vi "State Description - HelperVI and Equivalent String.vi"() -> ()   [LabVIEW 2014]
uses:
  user.lib/_NEVSTOP/JKI State Machine ++/JKI-State-Machine-Plus.lvlib
panel:
  out "Equivalent String (Broadcast Message with Argument)":string="Status Changed >> Argument-> <all>"
  out "Equivalent String (Broadcast Message)":string="Status Changed-> <all>"
  out "Equivalent String (Async Message)":string="State >> Argument->DestModuleName"
  out "Equivalent String (Sync Message)":string="State >> Argument@DestModuleName"
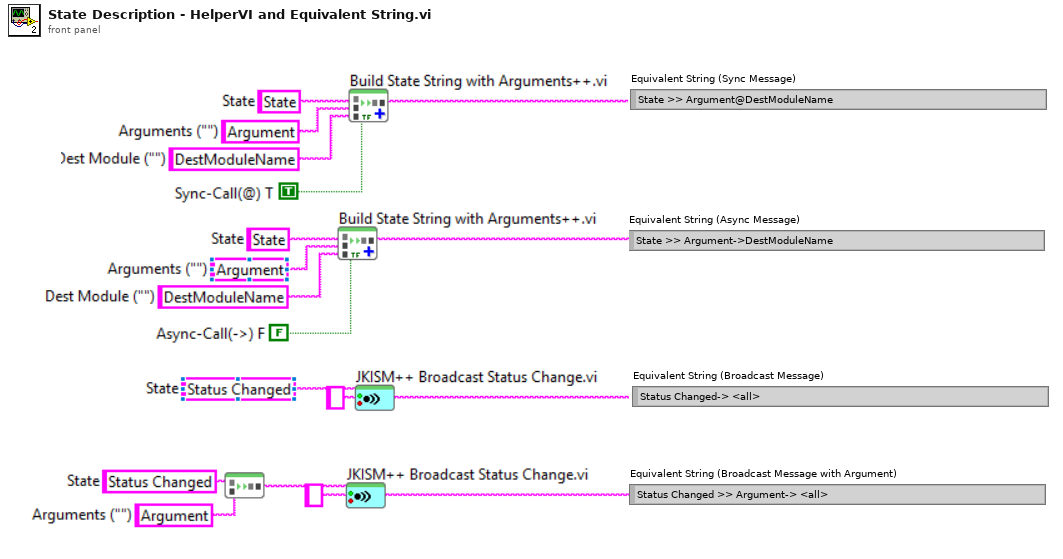
[diagram p1: front panel]
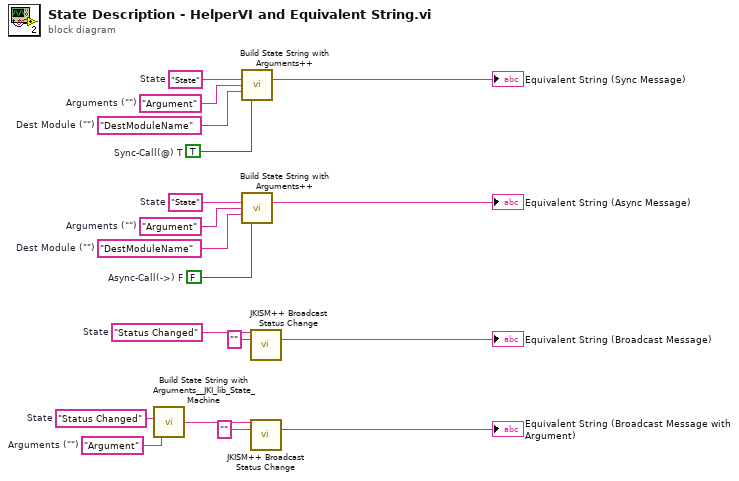
[diagram p0: block diagram]
diagram:
  w3 = "Argument"  # Arguments ("")
  w2 = "Status Changed"  # State
  w8 = "Status Changed"  # State
  w9 = FALSE  # Async-Call(->) F
  w11 = "Argument"  # Arguments ("")
  w12 = "DestModuleName"  # Dest Module ("")
  w10 = "State"  # State
  w15 = TRUE  # Sync-Call(@) T
  w17 = "Argument"  # Arguments ("")
  w16 = "DestModuleName"  # Dest Module ("")
  w18 = "State"  # State
  n1 = call <vilib>:"Build State String with Arguments__JKI_lib_State_Machine.vi"("Arguments (\"\")"=w3, "State"=w2) -> ("State with Arguments"=w1:string)  [unwired: 4 in]
  n2 = call "Build State String with Arguments++.vi"("State"=w18, "Arguments (\"\")"=w17, "Dest Module (\"\")"=w16, "Sync-Call(@) T By Default/Async-Call(->) F"=w15) -> ("State with Arguments"=→"Equivalent String (Sync Message)":string)  [unwired: 11 in]
  n3 = call "Build State String with Arguments++.vi"("State"=w10, "Arguments (\"\")"=w11, "Dest Module (\"\")"=w12, "Sync-Call(@) T By Default/Async-Call(->) F"=w9) -> ("State with Arguments"=→"Equivalent String (Async Message)":string)  [unwired: 11 in]
  n4 = call "JKISM++ Broadcast Status Change.vi"("Status with Arguments"=w8, "State(s) in (\"\")"="" ("State(s) in (\"\")")) -> ("States Out"=→"Equivalent String (Broadcast Message)":string)  [unwired: 13 in]
  n5 = call "JKISM++ Broadcast Status Change.vi"("Status with Arguments"=w1, "State(s) in (\"\")"="" ("State(s) in (\"\")")) -> ("States Out"=→"Equivalent String (Broadcast Message with Argument)":string)  [unwired: 13 in]
